vi "PJT_01.vi"() -> ()   [LabVIEW 2019]
uses:
  <vilib>/express/express shared/transition.llb/Dynamic To Waveform Array.vi
  <vilib>/express/express arith-compare/Formula/Block/exnFormulaBlock how many pts in the wave.vi
  <vilib>/express/express shared/ex_Modify Signal Name.vi
  <vilib>/express/express shared/transition.llb/Waveform Array To Dynamic.vi
  <vilib>/express/express arith-compare/Formula/XNode/ExpressFormulaBlockNode.xnode
panel:
  out "불리언":bool
  in  "정지":bool
  out "웨이브폼 그래프":dynamicdata(graph)
  in  "노브":dbl(knob) scale=0.0..10.0
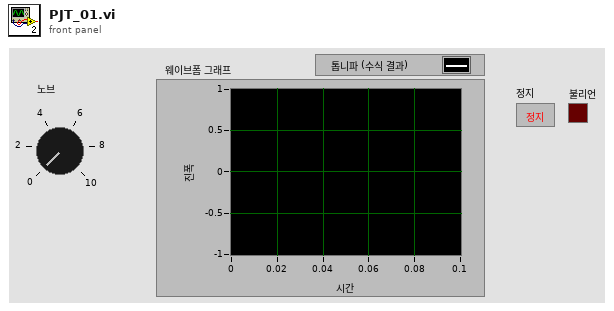
[diagram p1: front panel]
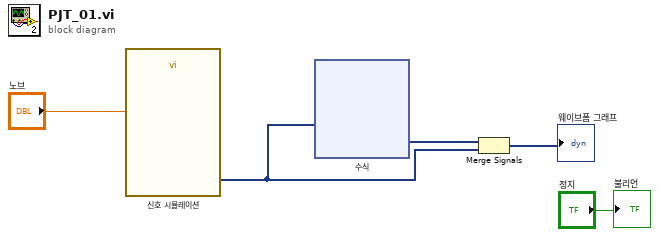
[diagram p0: block diagram]
diagram:
  n1 = call "신호 시뮬레이션"("Amplitude"="노브") -> ("톱니파"=w2:dynamicdata)  [unwired: 13 in, 1 out]
  n2 = xnode "수식"("톱니파"=w2) -> ("결과"=w3:dynamicdata)  [unwired: 1 in, 1 out]
  n3 = Merge Signals(w3, w2) -> (→"웨이브폼 그래프":dynamicdata)
  "불리언" <- "정지"
